vi "Estimate_Threshold_Val_[Russel,2009].vi"(1 "[IN] Threshold Initial":u16, 2 "[IN] 1D Sort Rever Img":u16[](array[numeric])) -> (0 "[OUT] Threshold Estimation":u16)   [LabVIEW 2020]
uses:
  <vilib>/Analysis/5stat.llb/RMS (DBL).vi
  <vilib>/Analysis/baseanly.llb/Mean (DBL).vi
  <vilib>/Analysis/NI_AALPro.lvlib
  <vilib>/Analysis/NI_AALBase.lvlib
panel:
  out "Threshold estimations":u16[](array[numeric])
  out "Derivatives":dbl[](array[numeric])
  out "Diff":dbl[](array[numeric])
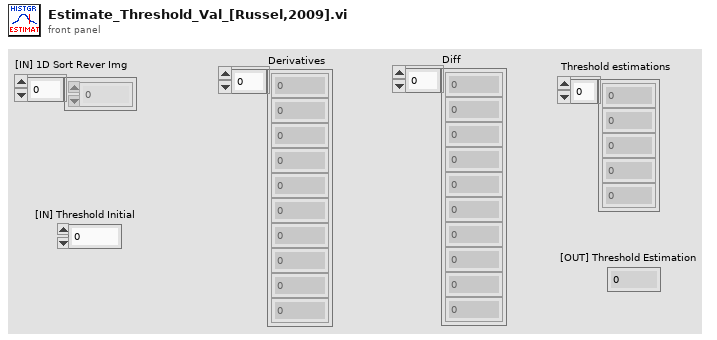
[diagram p1: front panel]
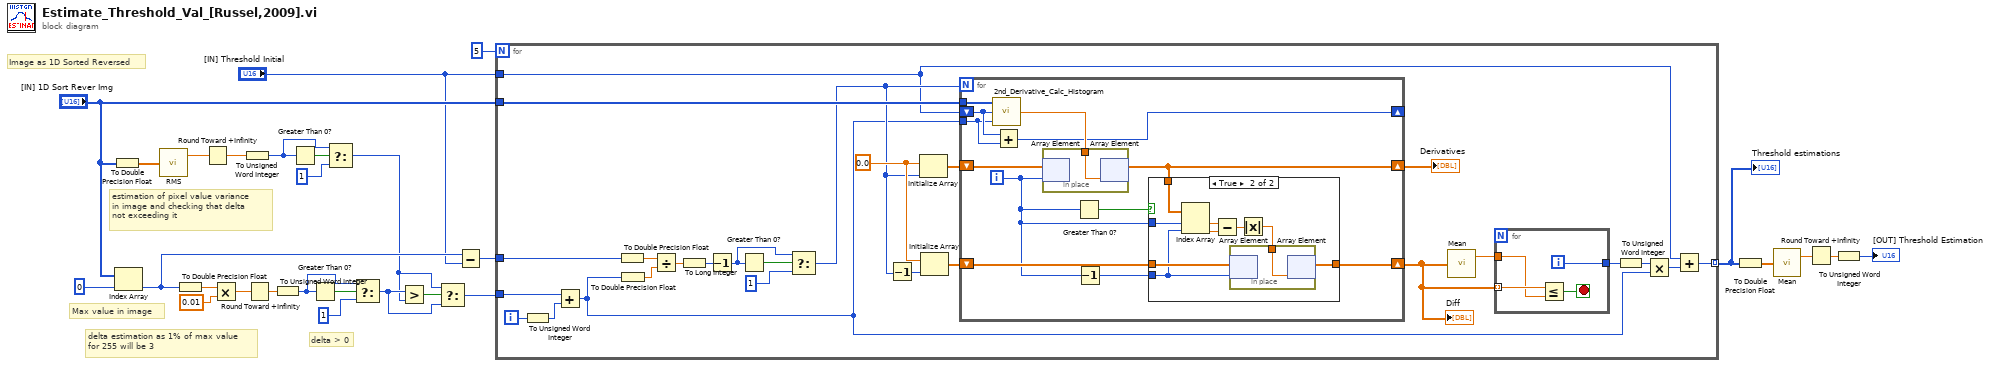
[diagram p0: block diagram]
diagram:
  # "estimation of pixel value variance \nin image and checking that delta\nnot exceeding it"
  # "delta > 0"
  # "delta estimation as 1% of max value\nfor 255 will be 3"
  # "Max value in image"
  # "Image as 1D Sorted Reversed"
  n1 = To Double Precision Float(number="[IN] 1D Sort Rever Img") -> (double precision float=w25:dbl[])
  n2 = Index Array(array="[IN] 1D Sort Rever Img", index=0) -> (element=w12:u16)
  n3 = call-poly <vilib>:"RMS.vi"("X"=w25) -> ("rms value"=w19:dbl)  [unwired: 1 out]
  n4 = To Double Precision Float(number=w12) -> (double precision float=w27:dbl)
  n5 = Round Toward +Infinity(x=w19) -> (ceil(x): smallest int >= x=w18:dbl)
  n6 = Multiply(x=w27, y=0.01) -> (x*y=w21:dbl)
  n7 = To Unsigned Word Integer(number=w18) -> (unsigned 16bit integer=w13:u16)
  n8 = Round Toward +Infinity(x=w21) -> (ceil(x): smallest int >= x=w20:dbl)
  n9 = To Unsigned Word Integer(number=w20) -> (unsigned 16bit integer=w23:u16)
  n10 = Greater Than 0?(x=w13) -> (x > 0?=w15:bool)
  n11 = Greater Than 0?(x=w23) -> (x > 0?=w24:bool)
  n12 = Select(t=w13, s=w15, f=u16 1) -> (s? t:f=w8:u16)
  n13 = Select(t=w23, s=w24, f=u16 1) -> (s? t:f=w16:u16)
  n14 = Greater?(x=w16, y=w8) -> (0:w17:bool)
  n15 = Select(t=w8, s=w17, f=w16) -> (s? t:f=w7:u16)
  n16 = Subtract(x=w12, y="[IN] Threshold Initial") -> (x-y=w11:u16)
  n17 = for {
    N: 5 -> [_]
    tunnel: w11 -> [w49]
    tunnel: "[IN] 1D Sort Rever Img" -> [w44]
    tunnel: "[IN] Threshold Initial" -> [w36]
    tunnel: w7 -> [w32]
    tunnel: [w35] -> w5 mode=indexing
    i -> [w34]
    w52 = 0.0 ("element")
    n18 = To Unsigned Word Integer(number=w34) -> (unsigned 16bit integer=w33:u16)
    n19 = Add(x=w32, y=w33) -> (x+y=w30:u16)
    n20 = To Double Precision Float(number=w49) -> (double precision float=w48:dbl)
    n21 = To Double Precision Float(number=w30) -> (double precision float=w47:dbl)
    n22 = Divide(x=w48, y=w47) -> (x/y=w46:dbl)
    n23 = To Long Integer(number=w46) -> (32bit integer=w45:i32)
    n24 = Decrement(x=w45) -> (x-1=w40:i32)
    n25 = Greater Than 0?(x=w40) -> (x > 0?=w43:bool)
    n26 = Select(t=w40, s=w43, f=1) -> (s? t:f=w41:i32)
    n27 = Decrement(x=w41) -> (x-1=w53:i32)
    n28 = Initialize Array(w52, w41) -> (w54:dbl[])
    n29 = Initialize Array(w52, w53) -> (w51:dbl[])
    n30 = for {
      N: w41 -> [_]
      tunnel: w44 -> [w70]
      tunnel: w30 -> [w66]
      shift-right: [w60] -> w50
      shift-left: w54 -> [w69]
      shift-right: [w65] -> _
      shift-left: w36 -> [w67]
      shift-right: [w62] -> w31
      shift-left: w51 -> [w63]
      i -> [w59]
      n31 = call "2nd_Derivative_Calc_Histogram.vi"("[IN] delta"=w66, "[IN] Threshold value"=w67, "[IN] 1D Sorted Reversed Img"=w70) -> ("[OUT] 2nd Derivative"=w68:dbl)  [unwired: 2 in]
      n32 = Add(x=w67, y=w66) -> (x+y=w65:u16)
      n33 = in-place {
        in-place-border: w68 -> [w82]
        n34 = in-place-array #1(w69, w59) -> ()  [unwired: 1 out]
        n35 = in-place-array #1(w82) -> (w60:dbl[])  [unwired: 1 out]
      }
      n36 = Greater Than 0?(x=w59) -> (x > 0?=w64:bool)
      n37 = Decrement(x=w59) -> (x-1=w61:i32)
      n38 = case shown="True" w64 {
        tunnel: w63 -> [w71 w80]
        tunnel: [w71 w79] -> w62
        tunnel: w61 -> [_ w76]
        tunnel: w60 -> [_ w78]
        tunnel: w59 -> [_ w77]
        frame False {
        }
        frame True {
          n39 = Index Array(array=w78, index #1=w77, index #2=w76) -> (element #1=w74:dbl, element #2=w73:dbl)
          n40 = Subtract(x=w74, y=w73) -> (x-y=w75:dbl)
          n41 = Absolute Value(x=w75) -> (abs(x)=w72:dbl)
          n42 = in-place {
            in-place-border: w72 -> [w81]
            n43 = in-place-array #2(w80, w76) -> ()  [unwired: 1 out]
            n44 = in-place-array #2(w81) -> (w79:dbl[])  [unwired: 1 out]
          }
        }
      }
    }
    "Diff" <- w31
    "Derivatives" <- w50
    n45 = call-poly <vilib>:"Mean.vi"("X"=w31) -> ("mean"=w29:dbl)  [unwired: 1 out]
    n46 = for {
      tunnel: w31 -> [w58] mode=indexing
      tunnel: w29 -> [w57]
      tunnel: [w55] -> w39
      i -> [w55]
      stop <- w56 stop-if-true
      n47 = Less Or Equal?(x=w58, y=w57) -> (x <= y?=w56:bool)
    }
    n48 = To Unsigned Word Integer(number=w39) -> (unsigned 16bit integer=w38:u16)
    n49 = Multiply(x=w38, y=w30) -> (x*y=w37:u16)
    n50 = Add(x=w36, y=w37) -> (x+y=w35:u16)
  }
  "Threshold estimations" <- w5
  n51 = To Double Precision Float(number=w5) -> (double precision float=w4:dbl[])
  n52 = call-poly <vilib>:"Mean.vi"("X"=w4) -> ("mean"=w3:dbl)  [unwired: 1 out]
  n53 = Round Toward +Infinity(x=w3) -> (ceil(x): smallest int >= x=w2:dbl)
  n54 = To Unsigned Word Integer(number=w2) -> (unsigned 16bit integer=→"[OUT] Threshold Estimation":u16)
